vi "Append Paragraphs.vi"(8 "error in (no error)":errorcluster, 9 "Styles":refnum<class "Style.lvclass">[](array[class]), 10 "Paragraphs":string[](array[string]), 11 "xwpfWriter in":refnum<class "xwpfWriter.lvclass">) -> (0 "error out":errorcluster, 3 "xwpfWriter out":refnum<class "xwpfWriter.lvclass">)   [LabVIEW 2017, in "LabVIEW NPOI.lvlib" / "xwpfWriter.lvclass"]
doc: "Appends <b>Paragraphs</b> formating as defined by <b>Styles</b> after the last paragraph within the document."
uses:
  xwpfWriter.lvclass
  Styles/Style/Style.lvclass
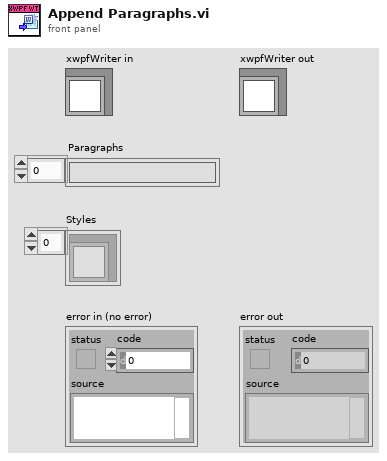
[diagram p1: front panel]
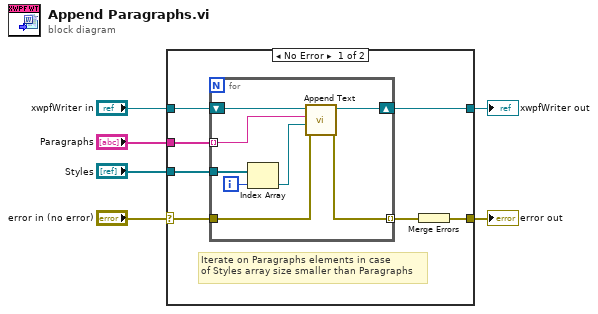
[diagram p0: block diagram]
diagram:
  n1 = case shown="No Error" "error in (no error)" {
    selector: "error in (no error)" -> [w9 w23]
    tunnel: [w7 w23] -> w5
    tunnel: [w12 w22] -> w3
    tunnel: "xwpfWriter in" -> [w13 w22]
    tunnel: "Paragraphs" -> [w11 _]
    tunnel: "Styles" -> [w10 _]
    frame No Error {
      # "Iterate on Paragraphs elements in case\nof Styles array size smaller than Paragraphs"
      n2 = for {
        shift-right: [w20] -> w12
        shift-left: w13 -> [w21]
        tunnel: w11 -> [w19] mode=indexing
        tunnel: w10 -> [w18]
        tunnel: w9 -> [w15]
        tunnel: [w14] -> w8 mode=indexing
        i -> [w17]
        n3 = Index Array(array=w18, index=w17) -> (element=w16:refnum<class "Style.lvclass">)
        n4 = call "Append Text.vi"("error in (no error)"=w15, "Style"=w16, "Text"=w19, "xwpfWriter in"=w21) -> ("error out"=w14:errorcluster, "xwpfWriter out"=w20:refnum<class "xwpfWriter.lvclass">)  [unwired: 6 in]
      }
      n5 = Merge Errors(w8) -> (w7:errorcluster)
    }
    frame Error {
    }
  }
  "error out" <- w5
  "xwpfWriter out" <- w3
